vi "Modbus Items - Check ranges.vi"(8 "error in (no error)":errorcluster, 11 "Modbus Items In":T1[](array[typedef])) -> (0 "error out":errorcluster, 3 "Modbus Items Out":T1[](array[typedef]))   [LabVIEW 2014, in "Modbus System Explorer.lvlib"]
doc: "This VI checks the following conditions:\n- All addresses defined stay within the 0-65535 address space.\n- For Read commands, per command, we respect the limit of 2000 coils or discrete inputs and 125 registers.\n- For Write commands, per command, we respect the limit of 1968 coils or 123 registers.\n\nAs soon as one of the condition is broken, an error is returned and VI execution stopped."
uses:
  Modbus System Explorer.lvlib
  XML Deserializer/XML VIs/API/Controls/Modbus_Items.ctl
  XML Deserializer/XML VIs/API/Controls/Modbus_Item_Type.ctl
  Shared/Modbus Shared.lvlib
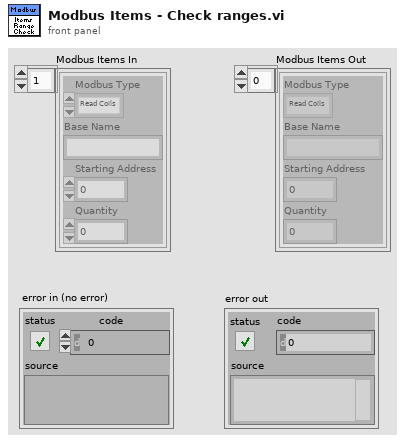
[diagram p1: front panel]
types:
  T1 = typedef "Modbus Shared.lvlib/Modbus_Items.ctl" = cluster{"Modbus Type":T2, "Base Name":string, "Starting Address":u16, "Quantity":u16}
  T2 = typedef "Modbus Shared.lvlib/Modbus_Item_Type.ctl" = enum16{"Read Coils", "Read Discrete Inputs", "Read Holding Registers", "Read Input Registers", "Write Multiple Coils", "Write Multiple Holding Registers", "Write Single Coil", "Write Single Holding Register", "Write Multiple Discrete Inputs", "Write Multiple Input Registers"}
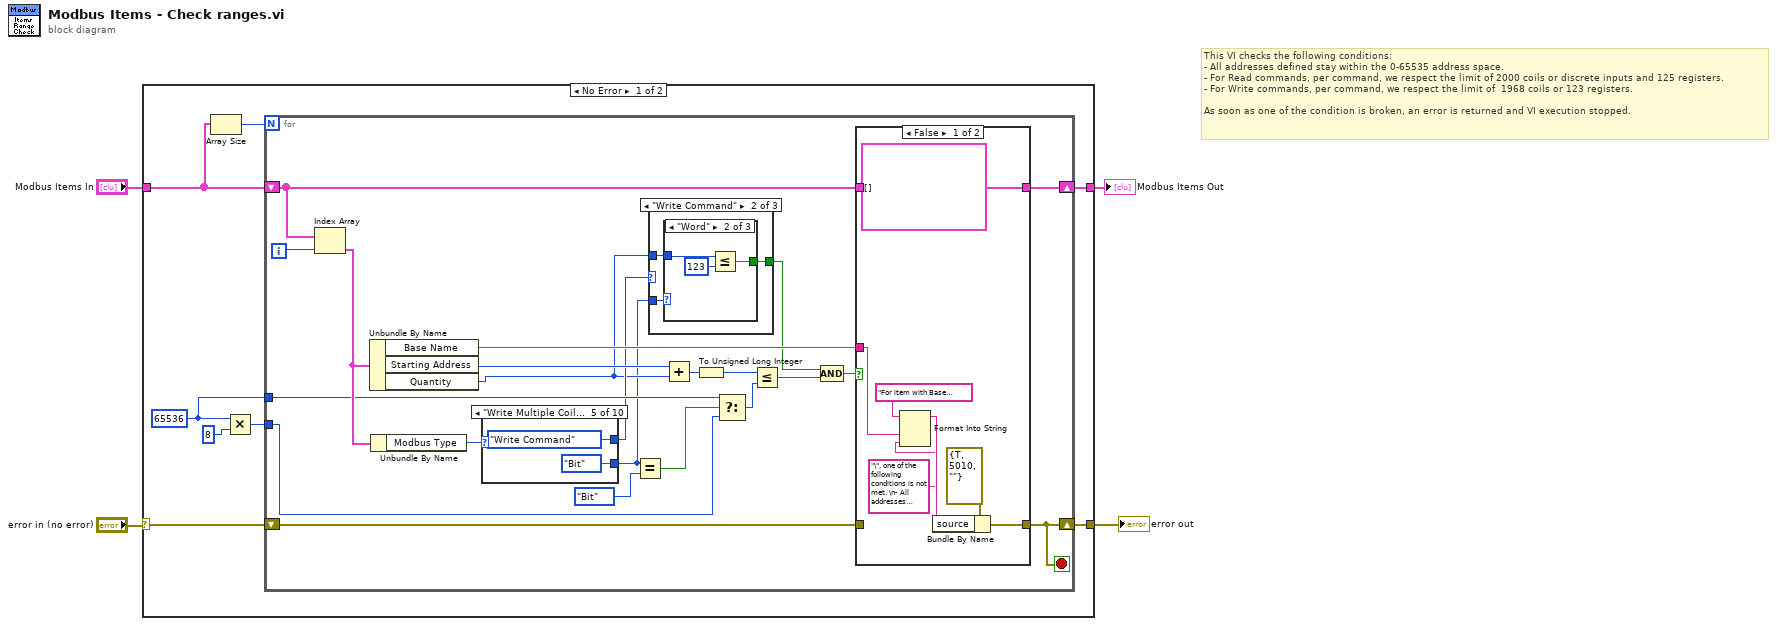
[diagram p0: block diagram]
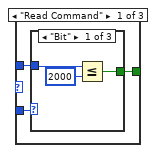
[diagram p2: hidden frame]
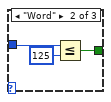
[diagram p3: hidden frame]
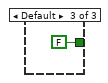
[diagram p4: hidden frame]
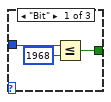
[diagram p5: hidden frame]
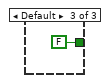
[diagram p6: hidden frame]
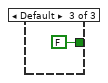
[diagram p7: hidden frame]
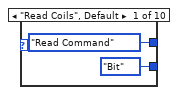
[diagram p9: hidden frame]
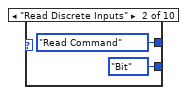
[diagram p10: hidden frame]
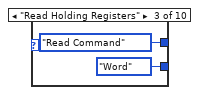
[diagram p11: hidden frame]
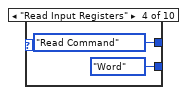
[diagram p12: hidden frame]
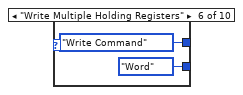
[diagram p13: hidden frame]
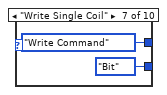
[diagram p14: hidden frame]
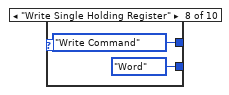
[diagram p15: hidden frame]
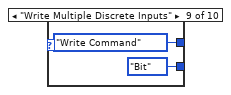
[diagram p16: hidden frame]
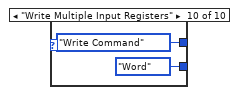
[diagram p17: hidden frame]
diagram:
  # "This VI checks the following conditions:\n- All addresses defined stay within the 0-65535 address space.\n- For Read commands, per command, we respect the limit of 2000 coils or discrete inputs and 125 registers.\n- For Write commands, per command, we respect the limit of  1968 coils or 123 registers.\n\nAs soon as one of the condition is broken, an error is returned and VI execution stopped."
  n1 = case shown="No Error" "error in (no error)" {
    selector: "error in (no error)" -> [w12 w86]
    tunnel: [w11 w86] -> w3
    tunnel: "Modbus Items In" -> [w5 w85]
    tunnel: [w10 w85] -> w1
    frame No Error {
      w8 = u32 65536
      n2 = Array Size(array=w5) -> (size(s)=w6:i32)
      n3 = Multiply(x=w8, y=u32 8) -> (x*y=w7:u32)
      n4 = for {
        N: w6 -> [_]
        shift-right: [w27] -> w11
        shift-left: w12 -> [w31]
        shift-right: [w29] -> w10
        shift-left: w5 -> [w30]
        tunnel: w8 -> [w19]
        tunnel: w7 -> [w20]
        i -> [w34]
        stop <- w27 stop-if-true
        n5 = Index Array(array=w30, index=w34) -> (element=w32:T1)
        n6 = Unbundle By Name(w32) -> ("Base Name"=w28:string, "Starting Address"=w26:u16, "Quantity"=w15:u16)
        n7 = Unbundle By Name(w32) -> ("Modbus Type"=w33:T2)
        n8 = case shown="\"Write Multiple Coils\"" w33 {
          tunnel: [enum16{"Read Command", "Write Command"}."Read Command" enum16{"Read Command", "Write Command"}."Read Command" enum16{"Read Command", "Write Command"}."Read Command" enum16{"Read Command", "Write Command"}."Read Command" enum16{"Read Command", "Write Command"}."Write Command" enum16{"Read Command", "Write Command"}."Write Command" enum16{"Read Command", "Write Command"}."Write Command" enum16{"Read Command", "Write Command"}."Write Command" enum16{"Read Command", "Write Command"}."Write Command" enum16{"Read Command", "Write Command"}."Write Command"] -> w16
          tunnel: [enum16{"Bit", "Word"}."Bit" enum16{"Bit", "Word"}."Bit" enum16{"Bit", "Word"}."Word" enum16{"Bit", "Word"}."Word" enum16{"Bit", "Word"}."Bit" enum16{"Bit", "Word"}."Word" enum16{"Bit", "Word"}."Bit" enum16{"Bit", "Word"}."Word" enum16{"Bit", "Word"}."Bit" enum16{"Bit", "Word"}."Word"] -> w14
          frame "Read Coils", Default {
          }
          frame "Read Discrete Inputs" {
          }
          frame "Read Holding Registers" {
          }
          frame "Read Input Registers" {
          }
          frame "Write Multiple Coils" {
          }
          frame "Write Multiple Holding Registers" {
          }
          frame "Write Single Coil" {
          }
          frame "Write Single Holding Register" {
          }
          frame "Write Multiple Discrete Inputs" {
          }
          frame "Write Multiple Input Registers" {
          }
        }
        n9 = Equal?(x=w14, y=enum16{"Bit", "Word"}."Bit") -> (x = y?=w21:bool)
        n10 = case shown="\"Write Command\"" w16 {
          tunnel: w15 -> [w36 w46 _]
          tunnel: w14 -> [w37 w47 _]
          tunnel: [w35 w45 FALSE] -> w13
          frame "Read Command" {
            n11 = case shown="\"Bit\"" w37 {
              tunnel: w36 -> [w40 w43 _]
              tunnel: [w38 w41 FALSE] -> w35
              frame "Bit" {
                n12 = Less Or Equal?(x=w40, y=u16 2000) -> (x <= y?=w38:bool)
              }
              frame "Word" {
                n13 = Less Or Equal?(x=w43, y=u16 125) -> (x <= y?=w41:bool)
              }
              frame Default {
              }
            }
          }
          frame "Write Command" {
            n14 = case shown="\"Word\"" w47 {
              tunnel: w46 -> [w50 w53 _]
              tunnel: [w48 w51 FALSE] -> w45
              frame "Bit" {
                n15 = Less Or Equal?(x=w50, y=u16 1968) -> (x <= y?=w48:bool)
              }
              frame "Word" {
                n16 = Less Or Equal?(x=w53, y=u16 123) -> (x <= y?=w51:bool)
              }
              frame Default {
              }
            }
          }
          frame Default {
          }
        }
        n17 = Add(x=w26, y=w15) -> (x+y=w24:u16)
        n18 = To Unsigned Long Integer(number=w24) -> (unsigned 32bit integer=w17:u32)
        n19 = Select(t=w19, s=w21, f=w20) -> (s? t:f=w18:u32)
        n20 = Less Or Equal?(x=w17, y=w18) -> (x <= y?=w23:bool)
        n21 = Compound Arithmetic op=AND(w13, w23) -> (w22:bool)
        n22 = case shown="False" w22 {
          tunnel: w31 -> [_ w63]
          tunnel: w30 -> [_ w64]
          tunnel: [T1[] [] ("Modbus Items In") w64] -> w29
          tunnel: w28 -> [w57 _]
          tunnel: [w61 w63] -> w27
          frame False {
            n23 = Format Into String(initial string="For item with Base Name \"" ("source"), w57, "\", one of the following conditions is not met. \n- All addresses defined stay within the 0-65535 address space.\n- For Read commands, per command, we respect the limit of 2000 coils or discrete inputs and 125 registers.\n- For Write commands, per command, we respect the limit of  1968 coils or 123 registers." ("source")) -> (resulting string=w58:string)  [unwired: 2 in, 1 out]
            n24 = Bundle By Name(cluster=errorcluster {"status"=TRUE, "code"=5010, "source"=""} ("error IO"), "source"=w58) -> (w61:errorcluster)
          }
          frame True {
          }
        }
      }
    }
    frame Error {
    }
  }
  "error out" <- w3
  "Modbus Items Out" <- w1
